vi "AsynchronousCall.vi"(8 "错误输入（无错误）":errorcluster, 10 "VI路径":path, 11 "类型说明符VI引用句柄（仅用于类型）":refnum<vi>) -> (0 "错误输出":errorcluster, 3 "引用输出":refnum<vi>)   [LabVIEW 2018]
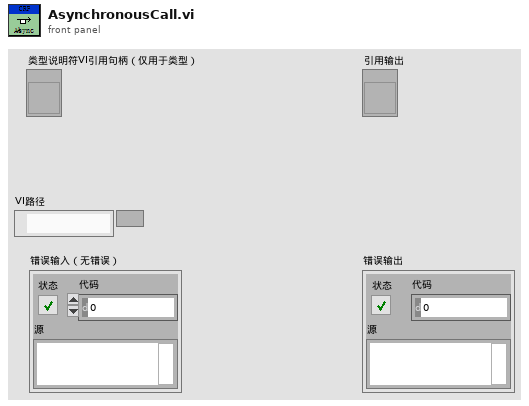
[diagram p1: front panel]
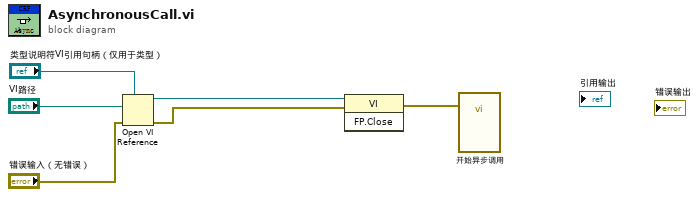
[diagram p0: block diagram]
diagram:
  n1 = Open VI Reference(type specifier VI Refnum (for type only)="类型说明符VI引用句柄（仅用于类型）", vi path="VI路径", error in (no error)="错误输入（无错误）") -> (vi reference=w3:refnum<vi>, error out=w2:errorcluster)  [unwired: 3 in]
  n2 = invoke class="VI" method="FP.Close"(reference=w3, error in=w2) -> (error out=w1:errorcluster)  [unwired: 1 in, 2 out]
  n3 = call-by-ref "开始异步调用"(error in=w1) -> ()  [unwired: 1 in, 2 out]
